vi "Real Eigenvalues and Vectors.vi"(3 "output option":T1=1 items=["Eigenvalues", "Eigenvalues & Vectors"], 4 "matrix type":i32(ring) items=["General", "Symmetric"], 5 "Input Matrix":T3) -> (0 "error":i32, 1 "Eigenvectors":T2, 2 "Eigenvalues":cdb[](array[numeric]))   [LabVIEW 2024, in "NI_AALPro.lvlib"]
doc: "<p>Finds the eigenvalues and right eigenvectors of the square <strong>Input Matrix</strong>. Wire data to the <strong>Input Matrix</strong> input to determine the polymorphic instance to use or <a href=\"nihelplauncher://docs/csh?context=lvcore_lvhowto_selectingdefaultinstpolyvi\">manually select</a> the instance.</p>"
uses:
  NI_AALPro.lvlib
  RealMatrix.ctl
  ComplexMatrix.ctl
  Eigenvalue and Vectors Output Option.ctl
  NI_AALBase.lvlib
  NI_Matrix.lvlib
panel:
  # "Eigenvalues and Vectors"
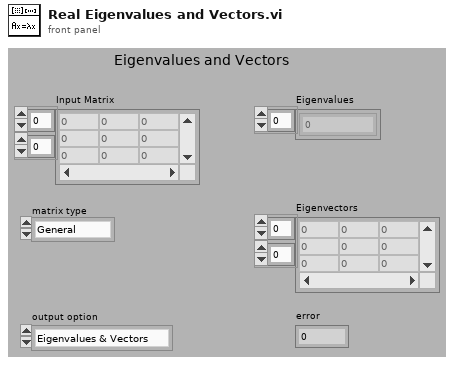
[diagram p1: front panel]
types:
  T1 = typedef "NI_AALPro.lvlib/Eigenvalue and Vectors Output Option.ctl" = i32
  T2 = typedef "NI_Matrix.lvlib/ComplexMatrix.ctl" = cdb[][]
  T3 = typedef "NI_Matrix.lvlib/RealMatrix.ctl" = dbl[][]
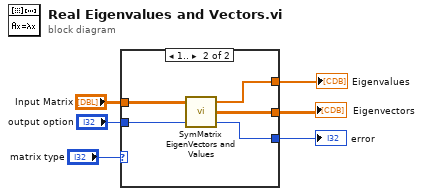
[diagram p0: block diagram]
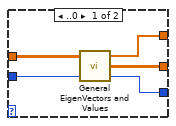
[diagram p2: hidden frame]
diagram:
  n1 = case shown="1.." "matrix type" {
    tunnel: "Input Matrix" -> [w11 w16]
    tunnel: "output option" -> [w7 w15]
    tunnel: [w10 w14] -> w5
    tunnel: [w9 w13] -> w4
    tunnel: [w8 w12] -> w3
    frame ..0 {
      n2 = call "General EigenVectors and Values.vi"("output option"=w7, "Input Matrix"=w11) -> ("error"=w8:i32, "Eigenvectors"=w9:T2, "Eigenvalues"=w10:cdb[])  [unwired: 1 in]
    }
    frame 1.. {
      n3 = call "SymMatrix EigenVectors and Values.vi"("Input Matrix"=w16, "output option"=w15) -> ("Eigenvalue"=w14:dbl[], "Eigenvector"=w13:T3, "error"=w12:i32)
    }
  }
  "Eigenvectors" <- w4
  "Eigenvalues" <- w5
  "error" <- w3
